vi "getDataCluster.vi"(8 "error in (no error)":errorcluster, 10 "Axis Letter":string, 11 "Controller in":refnum<class "Controller.lvclass">) -> (0 "error out":errorcluster, 2 "Information":T1, 3 "Controller out":refnum<class "Controller.lvclass">)   [LabVIEW 2019, in "Controller.lvclass"]
uses:
  Controller.lvclass
  Axis/Axis.lvclass
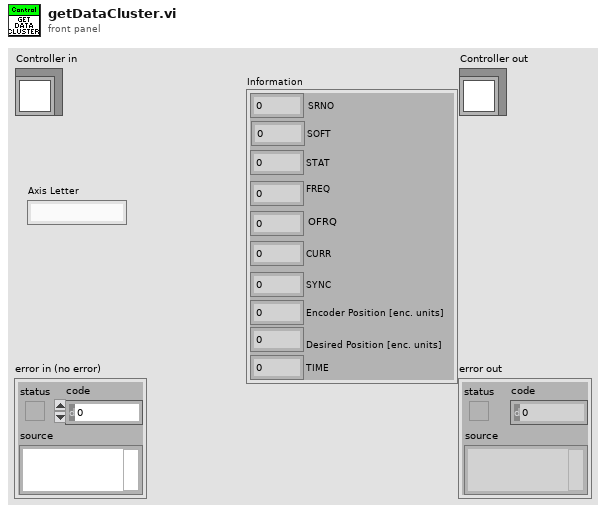
[diagram p1: front panel]
types:
  T1 = cluster{"SRNO":dbl, "SOFT":dbl, "STAT":dbl, "FREQ":dbl, "OFRQ":dbl, "CURR":dbl, "SYNC":dbl, "Encoder Position [enc. units]":dbl, "Desired Position [enc. units]":dbl, "TIME":dbl}
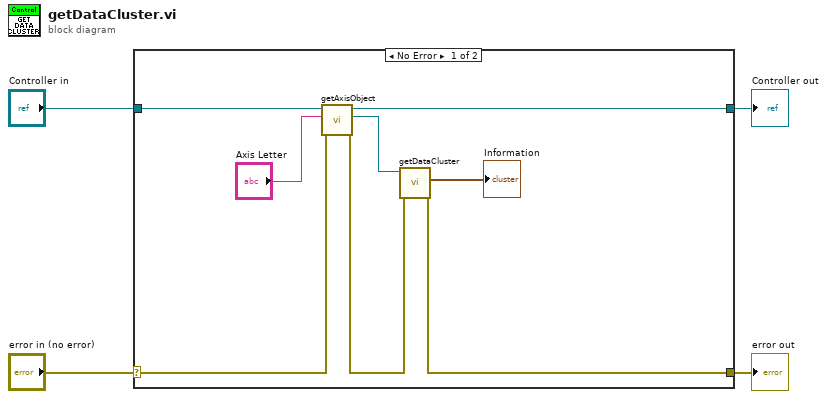
[diagram p0: block diagram]
diagram:
  n1 = case shown="No Error" "error in (no error)" {
    selector: "error in (no error)" -> [w7 w14]
    tunnel: [w11 w14] -> w3
    tunnel: [w10 w13] -> w1
    tunnel: "Controller in" -> [w12 w13]
    frame No Error {
      n2 = call-dynamic "getAxisObject.vi"("error in (no error)"=w7, "Axis Letter"="Axis Letter", "Controller in"=w12) -> ("error out"=w6:errorcluster, "Axis Object"=w5:refnum<class "Axis.lvclass">, "Controller out"=w10:refnum<class "Controller.lvclass">)  [unwired: 6 in]
      n3 = call-dynamic "getDataCluster.vi"("error in (no error)"=w6, "Axis in"=w5) -> ("error out"=w11:errorcluster, "Information"=→"Information":T1)  [unwired: 7 in, 1 out]
    }
    frame Error {
    }
  }
  "error out" <- w3
  "Controller out" <- w1
